vi "ProgG_002_MG.vi"() -> ()   [LabVIEW 2021]
uses:
  <vilib>/Utility/file.llb/Write Delimited Spreadsheet (DBL).vi
  <vilib>/Utility/file.llb/Read Delimited Spreadsheet (DBL).vi
panel:
  out "Odczytana tablica":dbl[](array[numeric])=[1.11, 2.22, 3.33, 4.44, 5.55]
  out "Czas zapsiu i odczytu [s]":ext=0.001
  in  "Tablica do zapisu":ext[](array[numeric])=[1.11, 2.22, 3.33, 4.44, 5.5500000000000000002]
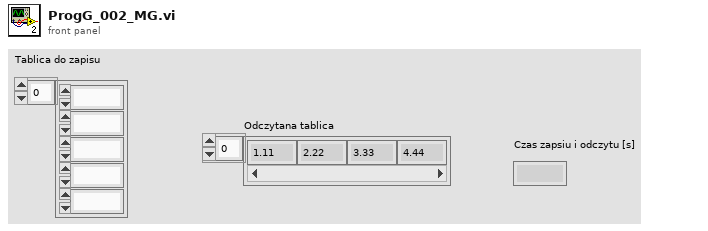
[diagram p1: front panel]
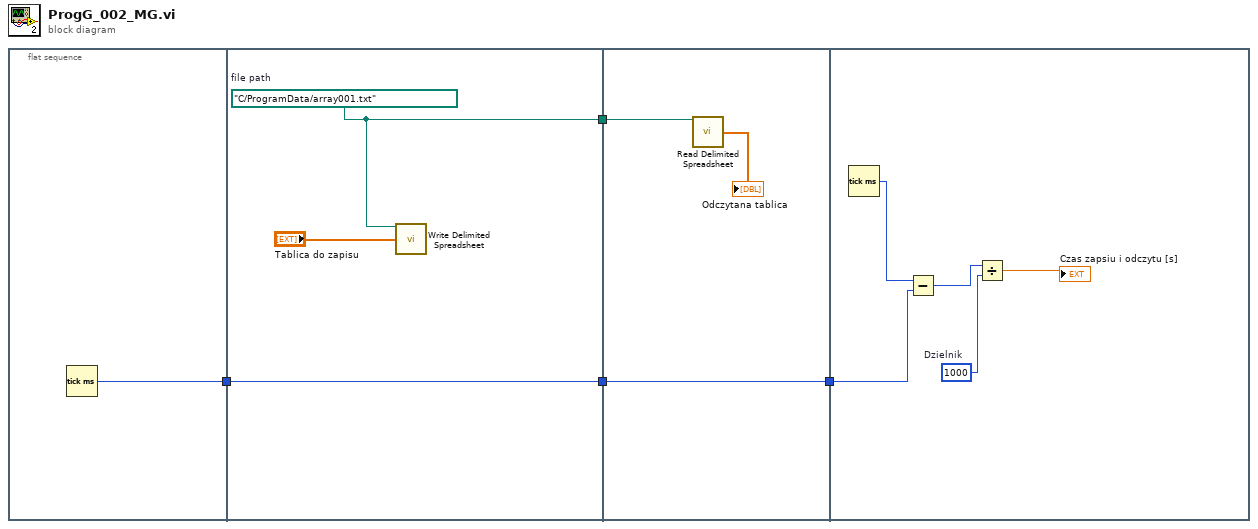
[diagram p0: block diagram]
diagram:
  n1 = flat-sequence {
    tunnel: [w5] -> w2
    tunnel: [w6] -> w3
    tunnel: w2 -> [w6]
    tunnel: [w7] -> w1
    tunnel: [w11] -> w4
    tunnel: w3 -> [w11]
    tunnel: w1 -> [w10]
    tunnel: w4 -> [w15]
    frame #0 {
      n2 = Tick Count (ms)() -> (millisecond timer value=w5:u32)
    }
    frame #1 {
      w7 = path "C:/ProgramData/array001.txt"  # file path
      n3 = call-poly <vilib>:"Write Delimited Spreadsheet.vi"("file path (dialog if empty)"=w7, "1D data"="Tablica do zapisu") -> ()  [unwired: 12 in, 2 out]
    }
    frame #2 {
      n4 = call-poly <vilib>:"Read Delimited Spreadsheet.vi"("file path (dialog if empty)"=w10) -> ("first row"=→"Odczytana tablica":dbl[])  [unwired: 9 in, 5 out]
    }
    frame #3 {
      w12 = u32 1000  # Dzielnik
      n5 = Tick Count (ms)() -> (millisecond timer value=w16:u32)
      n6 = Subtract(x=w16, y=w15) -> (x-y=w14:u32)
      n7 = Divide(x=w14, y=w12) -> (x/y=→"Czas zapsiu i odczytu [s]":dbl)
    }
  }
